vi "运动学正解.vi"(0 "正运动学输入":dbl[](array[numeric])=[0.0, 0.0, 0.0, 0.0, 0.0, 0.0], 1 "关节数":dbl=6.0) -> (2 "Tx":T1=[[3.102346606653217e-13, -1.0341155355510722e-13, -1.0, -2177.0], [1.0341155355510722e-13, 1.0, -1.0341155355507514e-13, -1.4612052517330483e-10], [1.0, -1.0341155355507514e-13, 3.102346606653324e-13, 558.0000000005964], [0.0, 0.0, 0.0, 1.0]] caption="实数矩阵" format="%#.4f", 3 "正解输出":dbl[](array[numeric])=[-2177.0, -1.4612052517330483e-10, 558.0000000005964, 1.0] format="%#.6f", 4 "腕部输出":dbl[](array[numeric])=[-2177.0, -1.4612052517330483e-10, 558.0000000005964])   [LabVIEW 2015]
uses:
  <vilib>/silver_ctls/ArrayMatrixCluster/Real Matrix NI_Silver.ctl
  <vilib>/Utility/file.llb/Read From Spreadsheet File (DBL).vi
  <vilib>/Analysis/Matrix/Numeric/Conversions/Array To Matrix - RA2.vi
  <vilib>/Analysis/Matrix/Numeric/Multiply/Multiply - RM,RM.vi
  <vilib>/Analysis/Matrix/NI_Matrix.lvlib
panel:
  in  "D-H参数表":dbl[][](array[numeric])=[[1.0, 0.0, 558.0, 0.0, 0.0], [2.0, 180.0, 0.0, 0.0, -90.0], [3.0, 90.0, 0.0, 764.0, 0.0], [4.0, 0.0, 993.0, 0.0, 90.0], [5.0, 0.0, 0.0, 0.0, -90.0], [6.0, 0.0, 420.0, 0.0, 90.0]]
  in  "机械臂长":dbl[](array[numeric])=[558.0, 764.0, 993.0, 420.0, 0.0, 0.0]
  in  "末端机械臂长":dbl=420.0
  in  "初始化矩阵":T1=[[1.0, 0.0, 0.0, 0.0], [0.0, 1.0, 0.0, 0.0], [0.0, 0.0, 1.0, 0.0], [0.0, 0.0, 0.0, 1.0]] caption="实数矩阵"
  out "Ti":dbl[][](array[numeric])=[[1.0, -0.0, 0.0, 0.0], [-0.0, -1.0341155355510722e-13, -1.0, -420.0], [0.0, 1.0, -1.0341155355510722e-13, -4.343285249314503e-11], [0.0, 0.0, 0.0, 1.0]] format="%#.4f"
  out "a":dbl
  out "d":dbl=420.0
  out "α":dbl=1.570796326795
  out "θ":dbl
  # "机械臂D-H参数表"
  # "θ"
  # "d"
  # "关节"
  # "a"
  # "α"
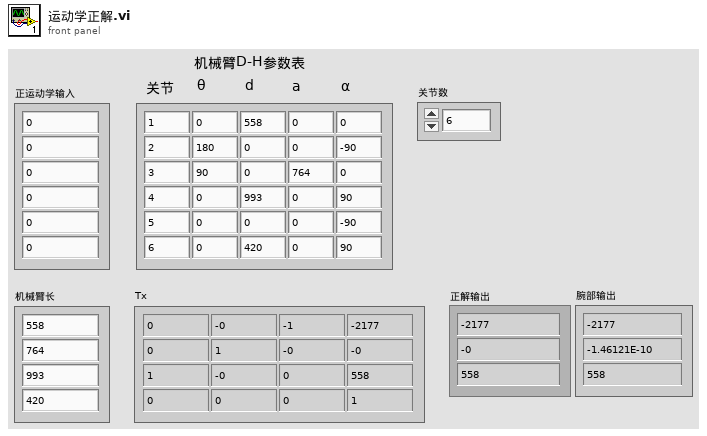
[diagram p1: front panel]
types:
  T1 = typedef "Real Matrix NI_Silver.ctl" = dbl[][]
  T2 = typedef "NI_Matrix.lvlib/RealMatrix.ctl" = dbl[][]
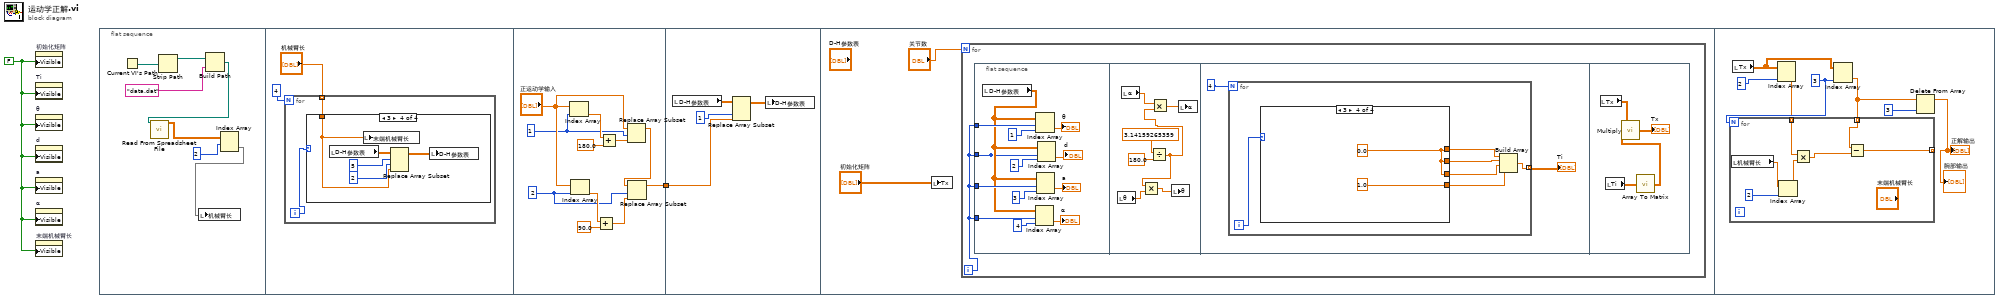
[diagram p0: block diagram]
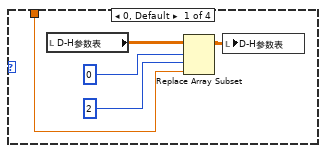
[diagram p2: hidden frame]
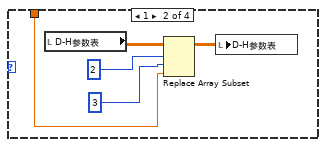
[diagram p3: hidden frame]
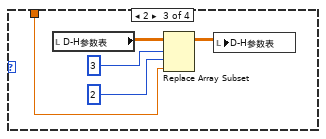
[diagram p4: hidden frame]
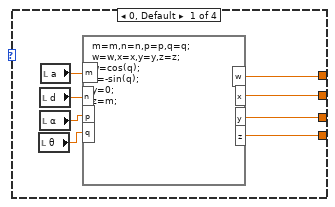
[diagram p5: hidden frame]
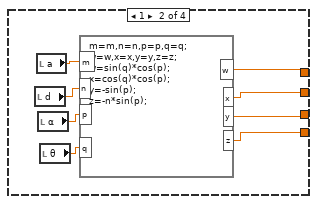
[diagram p6: hidden frame]
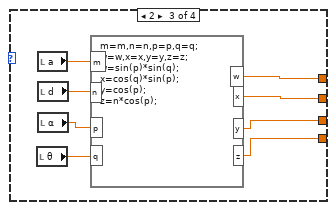
[diagram p7: hidden frame]
diagram:
  w2 = FALSE
  n1 = property on="初始化矩阵" class="Arr (严格)"("Visible"=w2) -> ()  [unwired: 2 in, 2 out]
  n2 = property on="Ti" class="Arr (严格)"("Visible"=w2) -> ()  [unwired: 2 in, 2 out]
  n3 = property on="θ" class="DigNum (严格)"("Visible"=w2) -> ()  [unwired: 2 in, 2 out]
  n4 = property on="d" class="DigNum (严格)"("Visible"=w2) -> ()  [unwired: 2 in, 2 out]
  n5 = property on="a" class="DigNum (严格)"("Visible"=w2) -> ()  [unwired: 2 in, 2 out]
  n6 = property on="α" class="DigNum (严格)"("Visible"=w2) -> ()  [unwired: 2 in, 2 out]
  n7 = property on="末端机械臂长" class="DigNum (严格)"("Visible"=w2) -> ()  [unwired: 2 in, 2 out]
  n8 = flat-sequence {
    tunnel: [w34] -> w1
    tunnel: w1 -> [w45]
    frame #0 {
      n9 = Current VI's Path() -> (path=w6:path)
      n10 = Strip Path(path=w6) -> (stripped path=w5:path)  [unwired: 1 out]
      n11 = Build Path(base path=w5, name or relative path="data.dat") -> (appended path=w3:path)
      n12 = call-poly <vilib>:"Read From Spreadsheet File.vi"("file path (dialog if empty)"=w3) -> ("all rows"=w9:dbl[][])  [unwired: 6 in, 4 out]
      n13 = Index Array(array=w9, index (row)=2) -> (element=w7:dbl[])  [unwired: 1 in]
      n14 = local write "机械臂长"(w7) -> ()
    }
    frame #1 {
      n15 = for {
        N: 4 -> [_]
        tunnel: "机械臂长" -> [w12] mode=indexing
        i -> [w13]
        n16 = case shown="3" w13 {
          tunnel: w12 -> [w15 w20 w25 w29]
          frame 0, Default {
            n17 = local read "D-H参数表"() -> (w18:dbl[][])
            n18 = Replace Array Subset(array=w18, new element=w15, index (row)=0, index (col)=2) -> (w14:dbl[][])
            n19 = local write "D-H参数表"(w14) -> ()
          }
          frame 1 {
            n20 = local read "D-H参数表"() -> (w23:dbl[][])
            n21 = Replace Array Subset(array=w23, new element=w20, index (row)=2, index (col)=3) -> (w19:dbl[][])
            n22 = local write "D-H参数表"(w19) -> ()
          }
          frame 2 {
            n23 = local read "D-H参数表"() -> (w28:dbl[][])
            n24 = Replace Array Subset(array=w28, new element=w25, index (row)=3, index (col)=2) -> (w24:dbl[][])
            n25 = local write "D-H参数表"(w24) -> ()
          }
          frame 3 {
            n26 = local read "D-H参数表"() -> (w33:dbl[][])
            n27 = local write "末端机械臂长"(w29) -> ()
            n28 = Replace Array Subset(array=w33, new element=w29, index (row)=5, index (col)=2) -> (w32:dbl[][])
            n29 = local write "D-H参数表"(w32) -> ()
          }
        }
      }
    }
    frame #2 {
      w36 = 2
      w38 = 1
      n30 = Index Array(array="正运动学输入", index=w38) -> (element=w44:dbl)
      n31 = Index Array(array="正运动学输入", index=w36) -> (element=w43:dbl)
      n32 = Add(x=w43, y=90.0) -> (x+y=w35:dbl)
      n33 = Add(x=w44, y=180.0) -> (x+y=w40:dbl)
      n34 = Replace Array Subset(array="正运动学输入", new element=w40, index=w38) -> (w37:dbl[])
      n35 = Replace Array Subset(array=w37, new element=w35, index=w36) -> (w34:dbl[])
    }
    frame #3 {
      n36 = local read "D-H参数表"() -> (w46:dbl[][])
      n37 = Replace Array Subset(array=w46, new element=w45, index (col)=1) -> (w48:dbl[][])  [unwired: 1 in]
      n38 = local write "D-H参数表"(w48) -> ()
    }
    frame #4 {
      n39 = local write "Tx"("初始化矩阵") -> ()
      n40 = for {
        N: "关节数" -> [_]
        i -> [w51]
        n41 = flat-sequence {
          tunnel: w51 -> [w64]
          tunnel: [w52] -> _
          tunnel: w51 -> [w63]
          tunnel: w51 -> [w61]
          tunnel: w51 -> [w52]
          frame #0 {
            n42 = local read "D-H参数表"() -> (w62:dbl[][])
            n43 = Index Array(array=w62, index (row)=w61, index (col)=4) -> (element=→"α":dbl)
            n44 = Index Array(array=w62, index (row)=w64, index (col)=1) -> (element=→"θ":dbl)
            n45 = Index Array(array=w62, index (row)=w63, index (col)=3) -> (element=→"a":dbl)
            n46 = Index Array(array=w62, index (row)=w52, index (col)=2) -> (element=→"d":dbl)
          }
          frame #1 {
            n47 = local read "θ"() -> (w69:dbl)
            n48 = local read "α"() -> (w67:dbl)
            n49 = Divide(x=3.14159265359, y=180.0) -> (x/y=w65:dbl)
            n50 = Multiply(x=w65, y=w69) -> (x*y=w68:dbl)
            n51 = Multiply(x=w67, y=w65) -> (x*y=w66:dbl)
            n52 = local write "θ"(w68) -> ()
            n53 = local write "α"(w66) -> ()
          }
          frame #2 {
            n54 = for {
              N: 4 -> [_]
              tunnel: [w74] -> w72 mode=indexing
              i -> [w75]
              n55 = case shown="3" w75 {
                tunnel: [w86 w93 w101 w105] -> w79
                tunnel: [w85 w90 w100 w105] -> w78
                tunnel: [w84 w89 w99 w105] -> w77
                tunnel: [w83 w88 w98 1.0] -> w76
                frame 0, Default {
                  n56 = local read "θ"() -> (w80:dbl)
                  n57 = local read "d"() -> (w82:dbl)
                  n58 = local read "α"() -> (w81:dbl)
                  n59 = local read "a"() -> (w87:dbl)
                  n60 = formula code="m=m,n=n,p=p,q=q;\nw=w,x=x,y=y,z=z;\nw=cos(q);\nx=-sin(q);\ny=0;\nz=m;"("m"=w87, "n"=w82, "p"=w81, "q"=w80) -> ("w"=w86:dbl, "x"=w85:dbl, "y"=w84:dbl, "z"=w83:dbl)
                }
                frame 1 {
                  n61 = local read "d"() -> (w94:dbl)
                  n62 = local read "a"() -> (w95:dbl)
                  n63 = local read "α"() -> (w92:dbl)
                  n64 = local read "θ"() -> (w91:dbl)
                  n65 = formula code="m=m,n=n,p=p,q=q;\nw=w,x=x,y=y,z=z;\nw=sin(q)*cos(p);\nx=cos(q)*cos(p);\ny=-sin(p);\nz=-n*sin(p);"("m"=w95, "n"=w94, "p"=w92, "q"=w91) -> ("w"=w93:dbl, "x"=w90:dbl, "y"=w89:dbl, "z"=w88:dbl)
                }
                frame 2 {
                  n66 = local read "θ"() -> (w96:dbl)
                  n67 = local read "a"() -> (w103:dbl)
                  n68 = local read "d"() -> (w102:dbl)
                  n69 = local read "α"() -> (w97:dbl)
                  n70 = formula code="m=m,n=n,p=p,q=q;\nw=w,x=x,y=y,z=z;\nw=sin(p)*sin(q);\nx=cos(q)*sin(p);\ny=cos(p);\nz=n*cos(p);"("m"=w103, "n"=w102, "p"=w97, "q"=w96) -> ("w"=w101:dbl, "x"=w100:dbl, "y"=w99:dbl, "z"=w98:dbl)
                }
                frame 3 {
                  w105 = 0.0
                }
              }
              n71 = Build Array(w79, w78, w77, w76) -> (w74:dbl[])
            }
            "Ti" <- w72
          }
          frame #3 {
            n72 = local read "Tx"() -> (w107:T1)
            n73 = local read "Ti"() -> (w109:dbl[][])
            n74 = call-poly <vilib>:"Array To Matrix.vi"("Real 2D Array"=w109) -> ("Real Matrix"=w108:T2)
            n75 = call-poly <vilib>:"Multiply.vi"("Real Matrix B"=w108, "Real Matrix A"=w107) -> ("A * B"=→"Tx":T2)
          }
        }
      }
    }
    frame #5 {
      w114 = 3
      n76 = local read "Tx"() -> (w115:T1)
      n77 = Index Array(array=w115, index (col)=2) -> (element=w113:dbl[])  [unwired: 1 in]
      n78 = Index Array(array=w115, index (col)=w114) -> (element=w112:dbl[])  [unwired: 1 in]
      n79 = for {
        N: w114 -> [_]
        tunnel: w113 -> [w123] mode=indexing
        tunnel: w112 -> [w122] mode=indexing
        tunnel: [w120] -> _ mode=indexing
        n80 = local read "机械臂长"() -> (w119:dbl[])
        n81 = Index Array(array=w119, index=2) -> (element=w117:dbl)
        n82 = Multiply(x=w123, y=w117) -> (x*y=w121:dbl)
        n83 = Subtract(x=w122, y=w121) -> (x-y=w120:dbl)
      }
      n84 = Delete From Array(array=w112, index=3) -> (array with subset deleted=→"正解输出" →"腕部输出":dbl[])  [unwired: 1 in, 1 out]
    }
  }
